vi "Exec Actions.vi"(10 "Trigger State":bool, 11 "TriggerAction Q in":refnum<class "TriggerAction Q.lvclass">) -> (3 "TriggerAction Q out":refnum<class "TriggerAction Q.lvclass">)   [LabVIEW 2016, in "TriggerAction Q.lvclass"]
uses:
  <userlib>/Common Components/TriggerAction Q/TriggerAction Q/TriggerAction Q.lvclass
  <userlib>/Common Components/TriggerAction Q/TriggerAction Q/TriggerAction Q.lvclass/TriggerAction Q.ctl
  <userlib>/Common Components/Function Messages/Action Dispatch Msg/Action Dispatch Msg.lvclass/Action Dispatch Msg.ctl
  <vilib>/ActorFramework/Message Enqueuer/Message Enqueuer.lvclass/Message Enqueuer.ctl
  <userlib>/Common Components/TriggerAction Q/TriggerAction Q/Element Data.ctl
  <vilib>/ActorFramework/Message Enqueuer/Enqueue.vi
  <userlib>/Common Components/Function Messages/Action Dispatch Msg/Action Dispatch Msg.lvclass
  C:/Program Files (x86)/National Instruments/LabVIEW 2016/vi.lib/ActorFramework/Message/Message.lvclass
  <vilib>/ActorFramework/Message Priority Queue/Priority Enqueue.vi
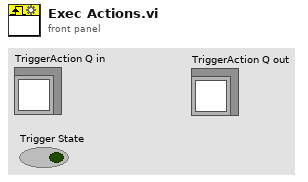
[diagram p1: front panel]
types:
  T1 = typedef "TriggerAction Q.lvclass/Element Data.ctl" = cluster{"Triggers":cluster{"Triggers for Array AND":string[]}[], "Actions":cluster{"Action Name":string, "Action Data":string}[]}
  T2 = cluster{"Action Name":string, "Action Data":string}[]
  T3 = cluster{"Action Name":string, "Action Data":string}
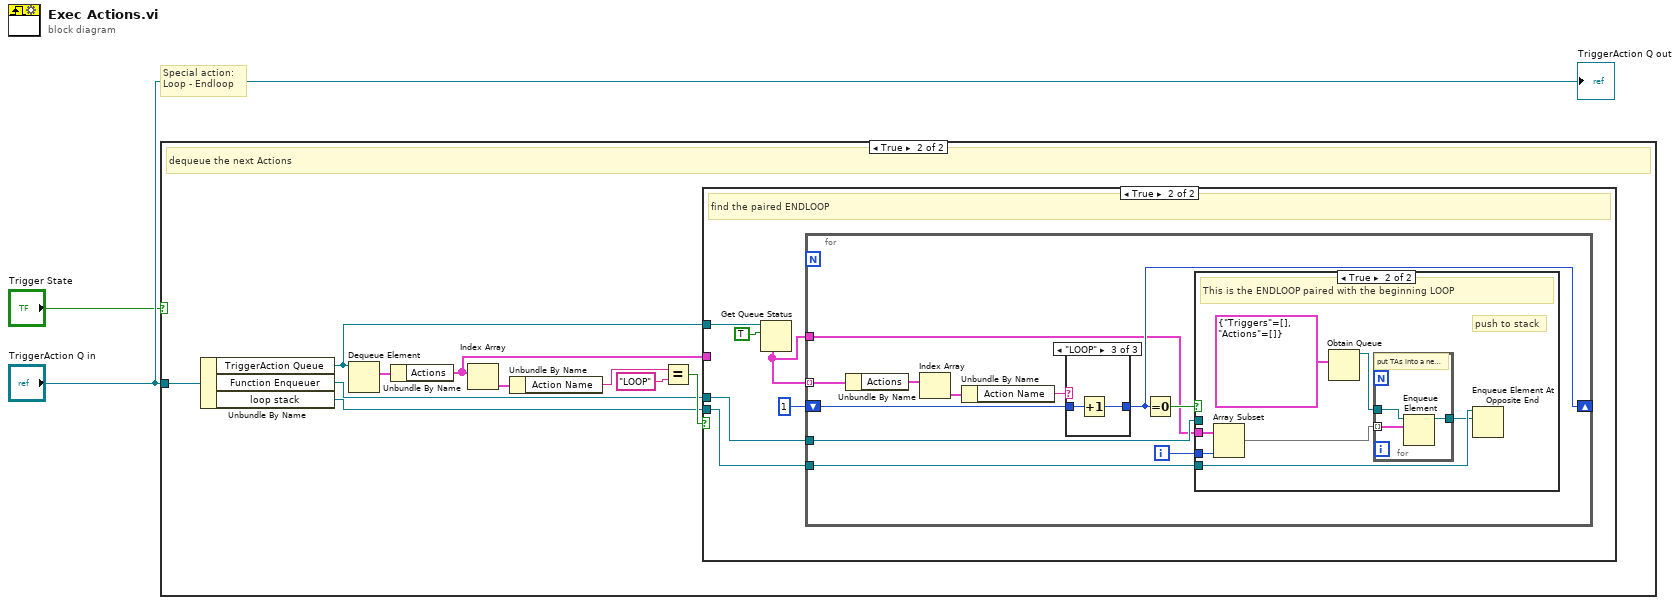
[diagram p0: block diagram]
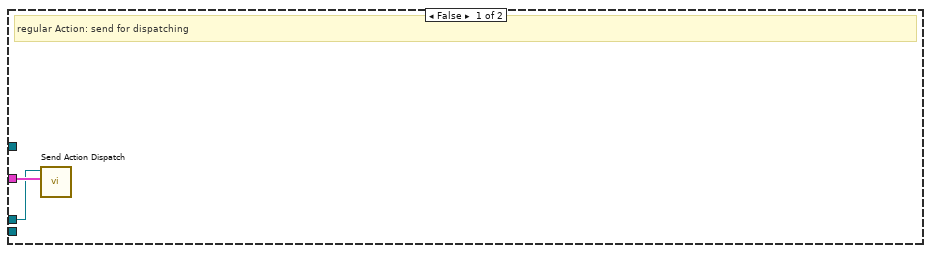
[diagram p3: hidden frame]
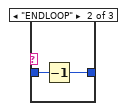
[diagram p6: hidden frame]
diagram:
  # "Special action:\nLoop - Endloop"
  n1 = case shown="True" "Trigger State" {
    tunnel: "TriggerAction Q in" -> [_ w12]
    frame False {
    }
    frame True {
      # "dequeue the next Actions"
      n2 = Unbundle By Name(w12) -> ("TriggerAction Queue"=w4:refnum<queue>, "Function Enqueuer"=w5:refnum<class "Message Enqueuer.lvclass">, "loop stack"=w3:refnum<queue>)
      n3 = Dequeue Element(queue=w4) -> (element=w11:T1)  [unwired: 2 in, 3 out]
      n4 = Unbundle By Name(w11) -> ("Actions"=w6:T2)
      n5 = Index Array(array=w6) -> (element=w10:T3)  [unwired: 1 in]
      n6 = Unbundle By Name(w10) -> ("Action Name"=w9:string)
      n7 = Equal?(x=w9, y="LOOP") -> (x = y?=w7:bool)
      n8 = case shown="True" w7 {
        tunnel: w6 -> [w14 _]
        tunnel: w5 -> [w13 w17]
        tunnel: w4 -> [_ w20]
        tunnel: w3 -> [_ w15]
        frame False {
          # "regular Action: send for dispatching"
          n9 = call <userlib>:"Send Action Dispatch.vi"("Actions"=w14, "Message Enqueuer"=w13) -> ()  [unwired: 8 in, 2 out]
        }
        frame True {
          # "find the paired ENDLOOP"
          n10 = Get Queue Status(queue=w20, return elements? (F)=TRUE) -> (elements=w16:T1[])  [unwired: 1 in, 7 out]
          n11 = for {
            tunnel: w16 -> [w31] mode=indexing
            shift-right: [w26] -> _
            shift-left: 1 -> [w27]
            tunnel: w17 -> [w24]
            tunnel: w16 -> [w23]
            tunnel: w15 -> [w21]
            i -> [w22]
            n12 = Unbundle By Name(w31) -> ("Actions"=w30:T2)
            n13 = Index Array(array=w30) -> (element=w29:T3)  [unwired: 1 in]
            n14 = Unbundle By Name(w29) -> ("Action Name"=w28:string)
            n15 = case shown="\"LOOP\"" w28 {
              tunnel: w27 -> [w42 w44 w46]
              tunnel: [w42 w43 w45] -> w26
              frame Default {
              }
              frame "ENDLOOP" {
                n16 = Decrement(x=w44) -> (x-1=w43:i32)
              }
              frame "LOOP" {
                n17 = Increment(x=w46) -> (x+1=w45:i32)
              }
            }
            n18 = Equal To 0?(x=w26) -> (x = 0?=w25:bool)
            n19 = case shown="True" w25 {
              tunnel: w24 -> [_ _]
              tunnel: w23 -> [_ w38]
              tunnel: w22 -> [_ w37]
              tunnel: w21 -> [_ w33]
              frame False {
              }
              frame True {
                # "push to stack"
                # "This is the ENDLOOP paired with the beginning LOOP"
                n20 = Array Subset(array=w38, length=w37) -> (w34:T1[])  [unwired: 1 in]
                n21 = Obtain Queue(element data type=T1 {"Triggers"=[], "Actions"=[]} ("Cluster")) -> (queue out=w35:refnum<queue>)  [unwired: 4 in, 2 out]
                n22 = for {
                  tunnel: w35 -> [w41]
                  tunnel: w34 -> [w40] mode=indexing
                  tunnel: [w39] -> w32
                  # "put TAs into a new queue"
                  n23 = Enqueue Element(queue=w41, element=w40) -> (queue out=w39:refnum<queue>)  [unwired: 2 in, 2 out]
                }
                n24 = Enqueue Element At Opposite End(queue=w33, element=w32) -> ()  [unwired: 2 in, 3 out]
              }
            }
          }
        }
      }
    }
  }
  "TriggerAction Q out" <- "TriggerAction Q in"
